vi "Flatten Measurements to String Array.vi"(11 "measurements":cluster{"Array":T1[]}[](array[cluster])) -> (3 "string array":string[][](array[string]))   [LabVIEW 2023, in "Logger.lvclass"]
uses:
  Logger.lvclass
  <vilib>/HPS-17000/MStream_grpc_CyclerMeasurement.ctl
  Logger.lvclass/Logger.ctl
  <vilib>/HPS-17000/NI_BC_client.lvlib
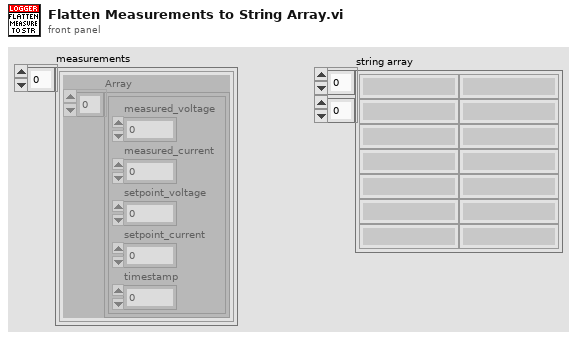
[diagram p1: front panel]
types:
  T1 = typedef "NI_BC_client.lvlib/MStream_grpc_CyclerMeasurement.ctl" = cluster{"measured_voltage":sgl, "measured_current":sgl, "setpoint_voltage":sgl, "setpoint_current":sgl, "timestamp":i64}
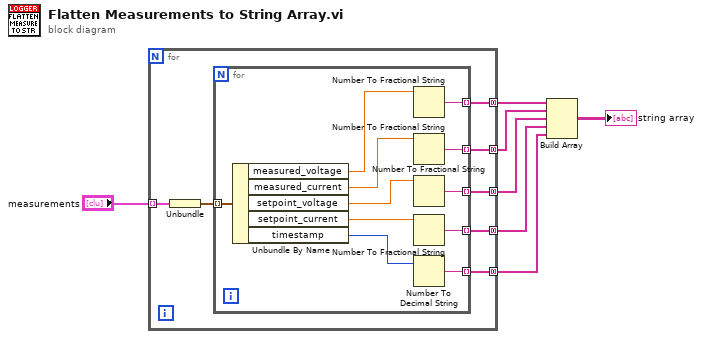
[diagram p0: block diagram]
diagram:
  n1 = for {
    tunnel: "measurements" -> [w10] mode=indexing
    tunnel: [w14] -> w3 mode=concatenating
    tunnel: [w13] -> w4 mode=concatenating
    tunnel: [w12] -> w5 mode=concatenating
    tunnel: [w11] -> w7 mode=concatenating
    tunnel: [w8] -> w6 mode=concatenating
    n2 = Unbundle(w10) -> ("Array"=w9:T1[])
    n3 = for {
      tunnel: w9 -> [w25] mode=indexing
      tunnel: [w18] -> w14 mode=indexing
      tunnel: [w19] -> w13 mode=indexing
      tunnel: [w20] -> w12 mode=indexing
      tunnel: [w15] -> w11 mode=indexing
      tunnel: [w17] -> w8 mode=indexing
      n4 = Unbundle By Name(w25) -> ("measured_voltage"=w24:sgl, "measured_current"=w23:sgl, "setpoint_voltage"=w22:sgl, "setpoint_current"=w21:sgl, "timestamp"=w16:i64)
      n5 = Number To Fractional String(number=w24) -> (F-format string=w17:string)  [unwired: 3 in]
      n6 = Number To Fractional String(number=w23) -> (F-format string=w18:string)  [unwired: 3 in]
      n7 = Number To Fractional String(number=w22) -> (F-format string=w19:string)  [unwired: 3 in]
      n8 = Number To Fractional String(number=w21) -> (F-format string=w20:string)  [unwired: 3 in]
      n9 = Number To Decimal String(number=w16) -> (decimal integer string=w15:string)  [unwired: 1 in]
    }
  }
  n10 = Build Array(w6, w3, w4, w5, w7) -> (→"string array":string[][])
